vi "GetProperties.vi"(8 "error in (no error)":errorcluster, 11 "Thing Info In":T2) -> (0 "error out":errorcluster, 2 "Array":string[][](array[string]), 3 "Thing Info Out":T2)   [LabVIEW 2015]
uses:
  <vilib>/httpClient/ClientHandle.ctl
  <vilib>/httpClient/LabVIEWHTTPClient.lvlib
panel:
  out "GET url":string
  out "ThingWorx Response":string
  out "result string":string
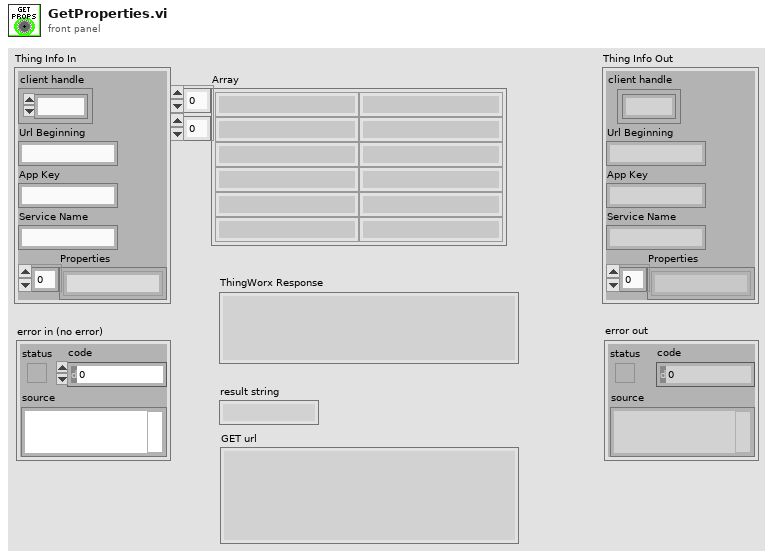
[diagram p1: front panel]
types:
  T1 = typedef "LabVIEWHTTPClient.lvlib/ClientHandle.ctl" = refnum<k1>
  T2 = cluster{"client handle":T1, "Url Beginning":string, "App Key":string, "Service Name":string, "Properties":string[]}
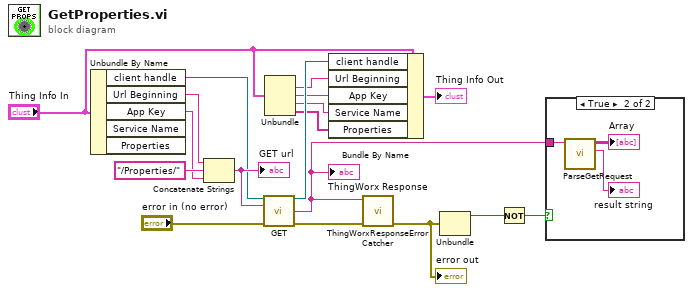
[diagram p0: block diagram]
diagram:
  n1 = Unbundle By Name("Thing Info In") -> ("client handle"=w13:T1, "Url Beginning"=w12:string, "App Key"=w11:string)  [unwired: 2 out]
  n2 = Concatenate Strings(w12, "/Properties/" ("url"), w11) -> (w16:string)
  "GET url" <- w16
  n3 = call <vilib>:"GET.vi"("client handle"=w13, "url"=w16, "error in (no error)"="error in (no error)") -> ("client handle out"=w9:T1, "body"=w3:string, "error out"=w2:errorcluster)  [unwired: 9 in, 1 out]
  "ThingWorx Response" <- w3
  n4 = Unbundle("Thing Info In") -> ("Url Beginning"=w7:string, "App Key"=w6:string, "Service Name"=w5:string, "Properties"=w4:string[])  [unwired: 1 out]
  n5 = Bundle By Name(cluster="Thing Info In", "client handle"=w9, "Url Beginning"=w7, "App Key"=w6, "Service Name"=w5, "Properties"=w4) -> (→"Thing Info Out":T2)
  n6 = call "ThingWorxResponseErrorCatcher.vi"("error in (no error)"=w2, "body"=w3) -> ("error out"=w1:errorcluster)  [unwired: 9 in]
  "error out" <- w1
  n7 = Unbundle(w1) -> ("status"=w15:bool)  [unwired: 2 out]
  n8 = Not(x=w15) -> (.not. x?=w14:bool)
  n9 = case shown="True" w14 {
    tunnel: w3 -> [_ w19]
    frame False {
    }
    frame True {
      n10 = call "ParseGetRequest.vi"("body"=w19) -> ("result string"=→"result string":string, "Array"=→"Array":string[][])  [unwired: 9 in]
    }
  }
